vi "NI-USB6343.vi"() -> ()   [LabVIEW 2020]
doc: "test"
uses:
  LabVIEW 2020 Toolkits/toolkits_lv2020_32bit/Synchronization.llb/SynchRefs_SetGet.ctl
  LabVIEW 2020 Toolkits/VI Server Toolkit/VI Server Libraries/VI Server_SetControl.llb/VI Server_BOOL_Set.vi
  LabVIEW 2020 Toolkits/VI Server Toolkit/VI Server Libraries/VI Server_Set Controls.llb/Set STR Control.vi
  LabVIEW 2020 Toolkits/VI Server Toolkit/VI Server Libraries/VI Server_GetControl.llb/VI Server_STR_Get.vi
  LabVIEW 2020 Toolkits/VI Server Toolkit/VI Server Libraries/VI Server_GetControl.llb/VI Server_DAQmx_Device_Get.vi
  LabVIEW 2020 Toolkits/VI Server Toolkit/VI Server Toolkit LV2013.lvlib
panel:
  in  "LastAction.AddToSecuence":bool
  out "System.Message":string caption="System Message"
  in  "Help":bool
  in  "FP.Hide":bool caption="FrontPanel.Hide"
  in  "EXIT":bool
  in  "Tab.Main":T1(tab)
  in  "AI.SaveGraphToFile":bool
  in  "AI.Graph.Plots":u16(ring) items=["NI-USB6343/ai0", "NI-USB6343/ai2"]
  out "AI.WaveformGraph":waveform(dbl)[](graph) caption="Waveform Graph"
  in  "AI.MultiChannelAcquisition":bool
  in  "AI.PhysicalChannel.Include":bool
  out "AI.ActualSampleRate":dbl=1000.0 caption="Actual Sample Rate" format="%0.2f"
  out "AI.Averaged.Mesurement":dbl caption="Averaged Mesurement" format="%0.4f V"
  in  "AI.Measure":bool caption="AI:Measure"
  in  "AI.Number.Of.Samples":i32=100 caption="Number Of Samples"
  in  "AI.SampleRate":dbl=1000.0 caption="Sample Rate" format="%0.0f Hz"
  in  "AI.MinInputLimit":dbl caption="Min Input Limit" min=-10.0 max=10.0 format="%0.3f V"
  in  "AI.MaxInputLimit":dbl caption="Max Input Limit" min=-10.0 max=10.0 format="%0.3f V"
  in  "AI.TerminalConfiguration":u16(ring)=65535 caption="Terminal Configuration" items=["default"=65535, "RSE"=10083, "NRSE"=10078, "Differential"=10106, "Pseudodifferential"=12529]
  in  "AI.Sample.Mode":u16(ring)=12522 caption="Sample Mode" items=["Finite Samples"=10178, "Continuous Samples"=10123]
  in  "AI.Physical.Channel":tag="Dev1/ai0" caption="Physical Channel"
  out "AO.Update.Time":u32 caption="AO Update Time" format="%.0f msec"
  in  "AO.GenerationMode":u16(ring) caption="Generation Mode" items=["Voltage DC", "Voltage Sine Wave Generation", "Voltage Triangle Wave Generation", "Voltage Square Wave Generation", "Voltage Sawtooth Wave Generation"]
  in  "AO.Physical.Channel":tag="Dev1/ai0" caption="Physical Channel"
  in  "AO.Update":bool
  in  "AO.Output":bool caption="AO:Output"
  in  "AO.SampleMode":u16(ring) caption="Sample Mode" items=["Finite Samples"=10178, "Continious Samples"=10123]
  in  "AO.NumberOfSamples":i32=1000 caption="Number Of Samples" min=2
  in  "AO.SampleRate":dbl=1000.0 caption="Sample Rate" format="%0.1f Hz"
  in  "AO.Sample.Clock.Source":tag="OnboardClock" caption="Sample Clock Source"
  out "AO.ActualSampleRate":dbl=1000.0 caption="Actual Sample Rate" format="%0.2f"
  in  "AO.MaxVoltage":dbl=5.0 caption="Max Voltage" format="%0.3f V"
  in  "AO.MinVoltage":dbl=-5.0 caption="Min Voltage" format="%0.3f V"
  out "AO.WaveformGraph":waveform(dbl)(graph) caption="Waveform Graph"
  in  "AO.OutputVoltage":dbl(slide) caption="Amplitude" min=-10.0 max=10.0 scale=-10.0..10.0 scale format="%0.3f V"
  in  "AO.SinewaveFrequency":dbl=10.0 caption="Sinewave Frequency" format="%0.2p Hz"
  in  "DO.Port.Mask.Apply":bool caption="DO:Port.Mask.Apply"
  in  "DO.Port.Lines.31:24.Mask":u8 caption="Port&Lines 31:24" format="%08b"
  in  "DO.Port.Lines.23:16.Mask":u8 caption="Port&Lines 23:16" format="%08b"
  in  "DO.Port.Lines.15:8.Mask":u8 caption="Port&Lines 15:8" format="%08b"
  in  "DO.Port.Lines.7:0.Mask":u8 caption="Port&Lines 7:0" format="%08b"
  out "DO.Port.State.Verify":bool caption="Verified"
  out "DO.Line.State.Verify":bool caption="Verified"
  in  "DO.Line.State":bool caption="State"
  in  "DO.Line":tag="Dev1/port0/line0:7" caption="Line"
  in  "DO.Line.Update":bool caption="Update:"
  in  "DO.Port.Update":bool caption="DO:Port.Update"
  in  "DO.Port.Lines.31:24":u8 caption="Port&Lines 31:24" format="%08b"
  in  "DO.Port.Lines.23:16":u8 caption="Port&Lines 23:16" format="%08b"
  in  "DO.Port.Lines.15:8":u8 caption="Port&Lines 15:8" format="%08b"
  in  "DO.Port.Lines.7:0":u8 caption="Port&Lines 7:0" format="%08b"
  in  "DO.Port":tag="Dev1/port0/line0:7" caption="Port"
  out "DI.Line.State":bool caption="State"
  in  "DI.Port.Update":bool caption="DI:Port.Update"
  out "DI.Port.Lines.24:31":u8 caption="Port&Lines 31:24" format="%08b"
  out "DI.Port.Lines.16:23":u8 caption="Port&Lines 23:16" format="%08b"
  out "DI.Port.Lines.8:15":u8 caption="Port&Lines 15:8" format="%.0b"
  out "DI.Port.Lines.0:7":u8 caption="Port&Lines 7:0" format="%08b"
  in  "DI.Port":tag="Dev1/port0/line0:7" caption="Port"
  in  "DI.Line":tag="Dev1/port0/line0:7" caption="Line"
  in  "DI.Line.Update":bool caption="Update:"
  out "ctr3.Out.Duty Cycle.Actual":dbl caption="Ctr3: Duty Cycle Actual" format="%.2f"
  out "ctr3.Out.Frequency.Actual":dbl caption="Ctr3: Frequency Actual" format="%0.3f Hz"
  out "ctr2.Out.Duty Cycle.Actual":dbl caption="Ctr2: Duty Cycle Actual" format="%.2f"
  out "ctr2.Out.Frequency.Actual":dbl caption="Ctr2: Frequency Actual" format="%0.3f Hz"
  out "ctr1.Out.Duty Cycle.Actual":dbl caption="Ctr1: Duty Cycle Actual" format="%.2f"
  out "ctr1.Out.Frequency.Actual":dbl caption="Ctr1: Frequency Actual" format="%0.3f Hz"
  out "ctr0.Out.Duty Cycle.Actual":dbl caption="Ctr0: Duty Cycle Actual" format="%.2f"
  out "ctr0.Out.Frequency.Actual":dbl caption="Ctr0: Frequency Actual" format="%0.3f Hz"
  in  "Cntr.Out.NumberOfPulses":i32=1000 caption="Number Of Pulses" min=1
  in  "Cntr.Out.Start":bool
  in  "Cntr.Out.Sample.Mode":u16(ring)=10123 caption="Sample Mode" items=["Finite Samples"=10178, "Continuous Samples"=10123, "Hardware Timed Single Point"=12522]
  in  "Cntr.Out.Duty.Cycle":dbl=0.5 caption="Duty Cycle" format="%.2f %"
  in  "Cntr.Out.Frequency":dbl=1.0 caption="Frequency" format="%0.3f Hz"
  in  "Cntr.Out.Output.Terminal":tag="/Dev1/PFI12" caption="Output Terminal"
  in  "Cntr.Out.Channel":tag="Dev1/ctr0" caption="Channel"
  out "ctr3.In.Count":u32 caption="Count.3:"
  out "ctr2.In.Count":u32 caption="Count.2:"
  out "ctr1.In.Count":u32 caption="Count.1:"
  out "ctr0.In.Count":u32 caption="Count.0:"
  in  "Cntr.In.Start":bool
  in  "Cntr.In.IntegrationTime":u32=10 format="%.0f msec"
  in  "Cntr.In.Sample.Clock.Source":tag="PFI0" caption="Sample Clock Source"
  in  "Cntr.In.ActiveEdge":u16(ring)=10280 caption="Active Edge" items=["Rising"=10280, "Falling"=10171]
  in  "Cntr.In.Input.Terminal":tag="PFI8" caption="Input.Terminal"
  in  "Cntr.In.Channel":tag="Dev1/port0/line0:7" caption="Channel Name"
  out "TestCase.Execute.All.Done":bool
  in  "Settings.Name.Remove":bool
  in  "Settings.Name.Add":bool
  in  "Settings.Name.New":string caption="Settings Name: New"
  in  "Settings.LOAD":bool
  in  "Settings.SAVE":bool
  in  "Settings.Name":u16(ring) caption="Label" items=["AI-NEW", "AO", "Counter In", "Counter Out", "Dig I/O"]
  in  "TestCase.Execute.Step.Pause":bool
  in  "TestCase.Execute.Steps":u16(ring) caption="Test Case: Pause Before Step" items=["1", "2", "3", "4", "5", "6", "7", "8", "9", "10"]
  in  "TestCase.Execute.ABORT":bool
  in  "TestCase.Execute.Next":bool
  in  "TestCase.Execute.Pause":bool
  out "TestCase.ExecutionTime":dbl caption="Execution Time:" format="%0.3f sec"
  in  "TestCase.Execution.StepTime":u32 caption="Seq. Execution: Step Time" format="%d msec"
  in  "TestCase.Execute.All":bool
  in  "TestCase.Execute.Selected":bool
  out "TestCase.SAVE.Success":bool
  in  "TestCase.SAVE":bool
  in  "SequenceFile.Open":bool
  in  "SequenceFile":path caption="Secuence File"
  in  "TestCaseConfiguration":i32[](listbox) caption="Test Case Configuration"
  in  "TestCase.StepDescription":string caption="Step Description:"
  in  "DisableFP_OpenOnIDN_Call":bool caption="Disable FP Open\nON *IDN? Call"
  in  "DisableFP_Hide":bool caption="Disable FP Hide"
  in  "UDP.Test.String1.SendLocal":bool caption="UDP.Test.String1.Send"
  in  "ProductType":string="USB-6343 (BNC)" caption="Product Type"
  in  "VI.WindowsTitle":string caption="Windows Title"
  in  "DAQmx.Device":tag caption="DAQmx: Device"
  in  "Cont.Measurements.CycleTime":u32 caption="Continius Measurements:\nCycleTime"
  in  "UDP.Test.String2.Send":bool
  in  "UDP.Test.String2":string caption="UDP: Test String 2"
  in  "UDP.Port.BC":u16=58433 caption="UDP: Port.BC"
  in  "UDP.Port.RT":u16=58432 caption="UDP: Port.RT"
  in  "UDP.LocalPort":u16=58434 caption="UDP: Local Port"
  in  "UDP.IP.Address":string="234.5.6.7" caption="UDP: IP Address"
  in  "UDP.Test.String1.Send.ToInstr":bool caption="UDP.Test.String1.Send"
  in  "UDP.Test.String1":string caption="UDP: Test String 1"
  in  "UDP.Responce.String.Monitor":bool
  out "UDP.ExecEng.Message.String":string caption="UDP: Execution Engine Message String"
  out "error out":errorcluster={"status"=TRUE, "code"=1055, "source"="Property Node in VI Server Toolkit LV2013.lvlib:VI server_Set Control Value from String Format.vi:5200001->DMM6500_UDP_ExecEng_Instruction_APPLY.vi->DMM6500_UDP_MAIN.vi->Keithley2100.vi"}
  in  "error in":errorcluster
  # "Important Note: Analog Input configuration shall\nstart from Physical Channel selection!"
  # "Important Note: Analog Output configuration shall\nstart from Physical Channel selection!"
  # "Analog Output Configuration (Generic)"
  # "Digital Output Port\nMASK"
  # "Instructions:\n1: Active Bit; 0: Masked Bit"
  # "Digital Output"
  # "Digital Input"
  # "Counter Input"
  # "Counter Input"
  # "Counter Output"
  # "M"
  # "M"
  # "Settings"
  # "M"
  # "M"
  # "Multicast IP addresses must be in the 224.0.0.0 to 239.255.255.255 range."
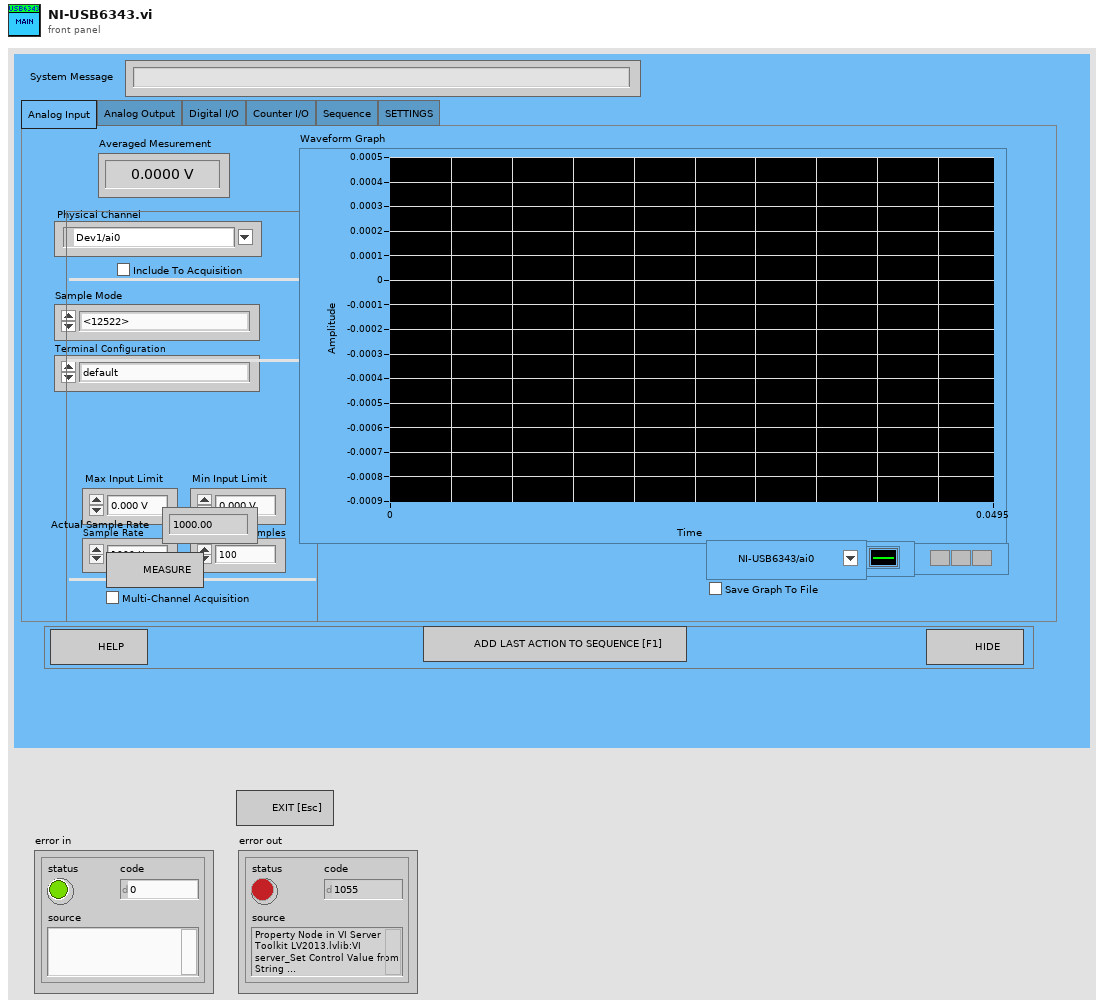
[diagram p1: front panel]
types:
  T1 = enum32{"Analog Input", "Analog Output", "Digital I/O", "Counter I/O", "Sequence", "SETTINGS"}
  T2 = typedef "VI Server_RefsCluster.ctl" = cluster{"Labels":string[], "Refs":refnum<vi>[], "VI Ref":refnum<vi>}
  T3 = typedef "SynchRefs_SetGet.ctl" = enum16{"Set", "Get"}
  T4 = enum8{"Enabled", "Disabled", "Disabled and Grayed Out"}
  T5 = cluster{"Color":u32, "PointStyle":u8, "LineStyle":u8, "Interp":u8, "LineWidth":u8, "BarPlotStyle":u8, "FillTo":i16, "XScaleIdx":u32, "YScaleIdx":u32, "Anti-Aliased":bool, "LabelFormat":u8, "TransitionType":u8, "TransitionLocation":u8, "DigitalLineStyle":u8}
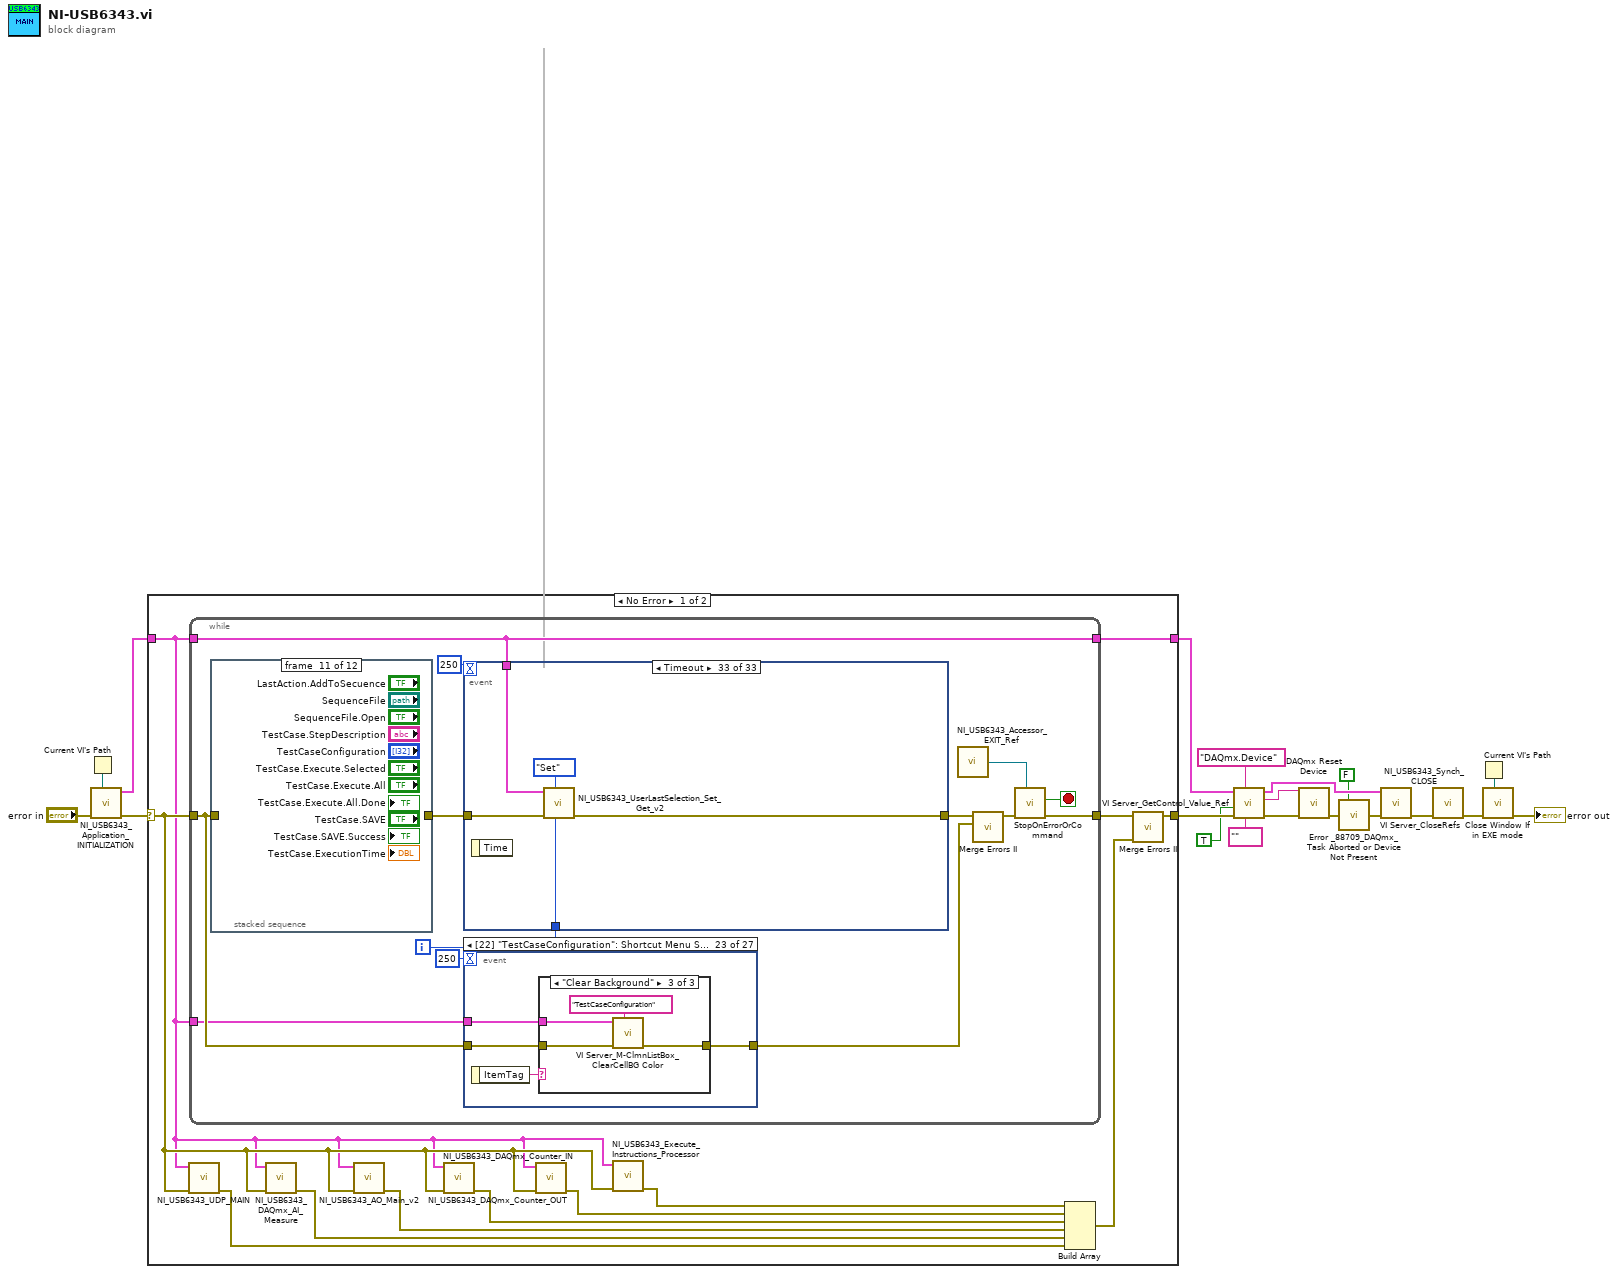
[diagram p0: block diagram]
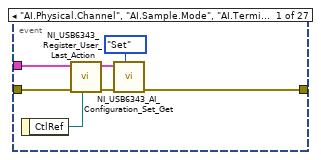
[diagram p2: hidden frame]
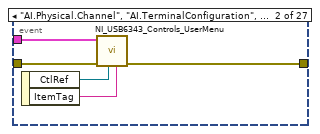
[diagram p3: hidden frame]
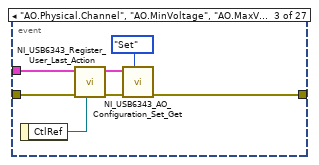
[diagram p4: hidden frame]
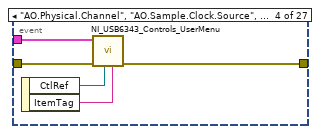
[diagram p5: hidden frame]
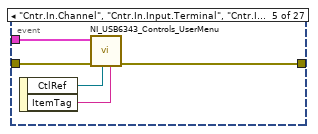
[diagram p6: hidden frame]
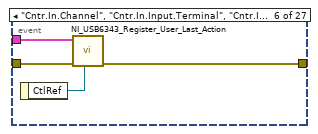
[diagram p7: hidden frame]
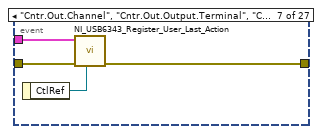
[diagram p8: hidden frame]
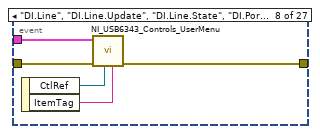
[diagram p9: hidden frame]
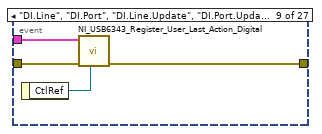
[diagram p10: hidden frame]
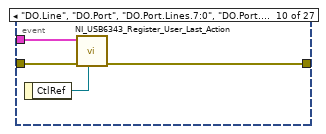
[diagram p11: hidden frame]
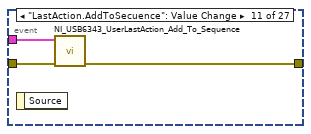
[diagram p12: hidden frame]
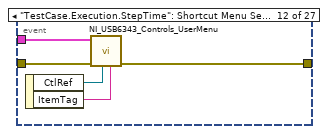
[diagram p13: hidden frame]
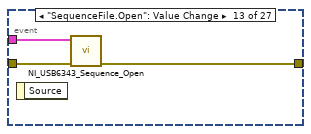
[diagram p14: hidden frame]
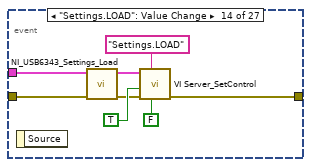
[diagram p15: hidden frame]
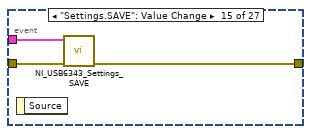
[diagram p16: hidden frame]
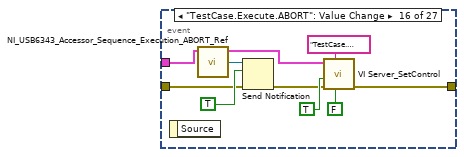
[diagram p17: hidden frame]
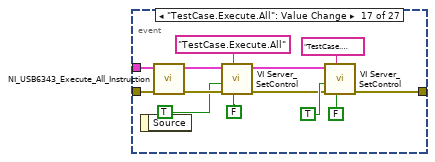
[diagram p18: hidden frame]
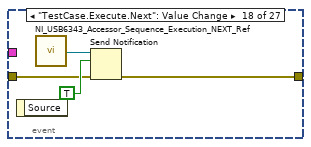
[diagram p19: hidden frame]
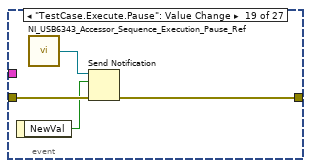
[diagram p20: hidden frame]
diagram:
  n1 = Current VI's Path() -> (path=w3:path)
  n2 = call "NI_USB6343_Application_INITIALIZATION.vi"("Top VI Path"=w3, "error in (no error)"="error in") -> ("error out"=w19:errorcluster, "VI Server Cluster.OUT"=w2:T2)  [unwired: 8 in]
  n3 = case shown="No Error" w19 {
    selector: w19 -> [w22 w407]
    tunnel: [w28 w407] -> w13
    tunnel: w2 -> [w20 w406]
    tunnel: [w31 w406] -> w11
    frame No Error {
      n4 = call "NI_USB6343_UDP_MAIN.vi"("error in (no error)"=w22, "VI Server.RefsCluster"=w20) -> ("error out"=w30:errorcluster)  [unwired: 9 in]
      n5 = while {
        tunnel: w22 -> [w36]
        tunnel: [w40] -> w29
        tunnel: w20 -> [w41]
        tunnel: [w41] -> w31
        tunnel: w20 -> [w32]
        i -> [w42]
        stop <- w39 stop-if-true
        n6 = stacked-sequence {
          tunnel: w36 -> [w405 _ _ _ _ _ _ _ _ _ _ _]
          tunnel: [w405 _ _ _ _ _ _ _ _ _ _ _] -> w44
          frame #0 {
          }
          frame #1 {
          }
          frame #2 {
          }
          frame #3 {
          }
          frame #4 {
          }
          frame #5 {
          }
          frame #6 {
          }
          frame #7 {
          }
          frame #8 {
          }
          frame #9 {
          }
          frame #10 {
          }
          frame #11 {
          }
        }
        n7 = event shown="[32] Timeout" {
          selector: _ -> [_ _ _ _ _ _ _ _ _ _ _ _ _ _ _ _ _ _ _ _ _ _ _ _ _ _ _ _ _ _ _ _ _]
          dyn-events: _ -> [_ _ _ _ _ _ _ _ _ _ _ _ _ _ _ _ _ _ _ _ _ _ _ _ _ _ _ _ _ _ _ _ _]
          timeout: 250 -> [_ _ _ _ _ _ _ _ _ _ _ _ _ _ _ _ _ _ _ _ _ _ _ _ _ _ _ _ _ _ _ _ _]
          tunnel: w44 -> [w187 w201 w204 w210 w219 w234 w241 w254 w266 w273 w276 w281 w292 w298 w304 w307 w311 w314 w318 w321 w325 w334 w341 w344 w345 w355 w357 w361 w372 w381 w390 w399 w403]
          tunnel: w42 -> [_ _ _ _ _ _ _ _ _ _ _ _ _ _ _ _ _ _ _ _ _ _ _ _ _ _ _ _ _ _ _ _ w402]
          tunnel: [w189 w199 w205 w212 w217 w232 w239 w251 w267 w271 w277 w279 w286 w297 w301 w306 w309 w312 w316 w319 w324 w331 w339 w342 w347 w350 w357 w359 w370 w379 w388 w397 w400] -> w35
          tunnel: w41 -> [w186 _ w206 w208 _ w230 w240 w253 w264 w272 w275 w280 w291 w296 w303 w305 w310 w313 _ w320 w323 _ w340 w343 _ w354 _ w358 _ w378 w387 w396 w401]
          event "AI.Physical.Channel": Value Change {
            n8 = event-data() -> ("OldVal"=w184:tag, "NewVal"=w182:tag)  [unwired: 1 in]
            n9 = call "NI_USB6343_AI_CheckPhysicalChannel.vi"("NewVal"=w182, "OldVal"=w184, "error in (no error)"=w187, "VI Server Cluster"=w186) -> ("error out"=w188:errorcluster, "AI.Settings.Update"=w183:bool, "VI Server Cluster DUP"=w185:T2)  [unwired: 5 in]
            n10 = case shown="True" w183 {
              tunnel: [w190 w193] -> w189
              tunnel: w188 -> [w190 w196]
              tunnel: w185 -> [_ w195]
              tunnel: w182 -> [_ w192]
              frame False {
              }
              frame True {
                n11 = Type Cast(x=w192) -> (*(type *) &x=w191:string)  [unwired: 1 in]
                n12 = call "NI_USB6343_AI_Configuration_Set_Get.vi"("SynchRefs.Set/Get"=SynchRefs_SetGet."Get", "error in (no error)"=w196, "VI Server Cluster"=w195) -> ("error out"=w194:errorcluster)  [unwired: 6 in, 2 out]
                n13 = property on="AI.WaveformGraph" class="WFGraph (strict)"(error in=w194, "Plot.Plot Name"=w191) -> (error out=w193:errorcluster)  [unwired: 1 in, 1 out]
              }
            }
          }
          event "AI.SaveGraphToFile": Value Change {
            n14 = event-data() -> ("NewVal"=w198:bool)  [unwired: 1 in]
            n15 = call "NI_USB6343_Accessor_AI_SaveGraphToFile_Ref.vi"() -> ("AI.SaveGraphToFile"=w200:refnum<notifier>)  [unwired: 6 in]
            n16 = Send Notification(notification=w198, notifier=w200, error in (no error)=w201) -> (error out=w199:errorcluster)  [unwired: 1 out]
          }
          event "AI.WaveformGraph": Plot Attribute Change {
            n17 = event-data() -> ("OldAttrib"=w203:T5, "NewAttrib"=w202:T5)  [unwired: 1 in]
            n18 = call "NI_USB6343_AI_Graph_PlotAttribute_ValueChanged.vi"("NewAttrib"=w202, "OldAttrib"=w203, "error in (no error)"=w204, "VI Server Cluster"=w206) -> ("error out"=w205:errorcluster)  [unwired: 7 in]
          }
          event "AO.GenerationMode": Value Change {
            n19 = event-data() -> ("NewVal"=w216:u16)  [unwired: 1 in]
            n20 = call "NI_USB6343_AO_Configuration_Set_Get.vi"("SynchRefs.Set/Get"=SynchRefs_SetGet."Set", "error in (no error)"=w210, "VI Server Cluster"=w208) -> ("error out"=w211:errorcluster, "VI Server Cluster.DUP"=w209:T2)  [unwired: 6 in, 1 out]
            n21 = call "NI_USB6343_AO_GenerationMode.vi"("AO.GenerationMode"=w216, "error in (no error)"=w211, "VI Server Cluster"=w209) -> ("error out"=w213:errorcluster)  [unwired: 7 in, 1 out]
            n22 = call "NI_USB6343_Accessor_ao_Waveform_Array_Update_Ref.vi"() -> ("ao.Waveform.Array.Update"=w215:refnum<notifier>)  [unwired: 6 in]
            n23 = Send Notification(notification=TRUE, notifier=w215, error in (no error)=w213) -> (error out=w212:errorcluster)  [unwired: 1 out]
          }
          event "AO.Output": Value Change {
            n24 = event-data() -> ("NewVal"=w218:bool)  [unwired: 1 in]
            n25 = disable-structure shown="Enabled" {
              disable-tunnel: w219 -> [w226 w227]
              disable-tunnel: w218 -> [w224 _]
              disable-tunnel: [w221 w227] -> w217
              frame Enabled {
                n26 = call "NI_USB6343_Accessor_ao0_State_Ref.vi"() -> ("ao0.State"=w225:refnum<notifier>)  [unwired: 6 in]
                n27 = Send Notification(notification=w224, notifier=w225, error in (no error)=w226) -> (error out=w222:errorcluster)  [unwired: 1 out]
                n28 = call "NI_USB6343_Accessor_ao_Waveform_Array_Update_Ref.vi"() -> ("ao.Waveform.Array.Update"=w223:refnum<notifier>)  [unwired: 6 in]
                n29 = Send Notification(notification=TRUE, notifier=w223, error in (no error)=w222) -> (error out=w221:errorcluster)  [unwired: 1 out]
              }
              frame Disabled {
              }
            }
          }
          event "AO.Physical.Channel": Value Change {
            n30 = event-data() -> ("NewVal"=w228:tag)  [unwired: 1 in]
            n31 = call "NI_USB6343_AO_Configuration_Set_Get.vi"("SynchRefs.Set/Get"=SynchRefs_SetGet."Get", "error in (no error)"=w234, "VI Server Cluster"=w230) -> ("error out"=w231:errorcluster, "VI Server Cluster.DUP"=w229:T2)  [unwired: 6 in, 1 out]
            n32 = call "NI_USB6343_AO_PhysicalChannel_UpdateGraph.vi"("AO.Physical.Channel"=w228, "error in (no error)"=w231, "VI Server Cluster"=w229) -> ("error out"=w232:errorcluster)  [unwired: 8 in]
          }
          event "AO.Sample.Clock.Source", "AO.SampleMode", "AO.SampleRate", "AO.NumberOfSamples", "AO.MaxVoltage", "AO.MinVoltage": Value Change {
            n33 = event-data() -> ()  [unwired: 1 in, 1 out]
            n34 = call "NI_USB6343_AO_ConfigurationAtributes.vi"("error in (no error)"=w241, "VI Server Cluster"=w240) -> ("error out"=w238:errorcluster)  [unwired: 8 in, 1 out]
            n35 = call "NI_USB6343_Accessor_ao0_State_Ref.vi"() -> ("ao0.State"=w236:refnum<notifier>)  [unwired: 6 in]
            n36 = Get Notifier Status(notifier=w236, error in (no error)=w238) -> (current notification=w235:bool, error out=w237:errorcluster)  [unwired: 3 out]
            n37 = case shown="True" w235 {
              tunnel: [w242 w247] -> w239
              tunnel: w237 -> [w242 w244]
              tunnel: w236 -> [_ w243]
              frame False {
              }
              frame True {
                w246 = TRUE ("notification")
                n38 = Send Notification(notification=FALSE, notifier=w243, error in (no error)=w244) -> (error out=w249:errorcluster)  [unwired: 1 out]
                n39 = call "NI_USB6343_Accessor_ao_Waveform_Array_Update_Ref.vi"() -> ("ao.Waveform.Array.Update"=w250:refnum<notifier>)  [unwired: 6 in]
                n40 = Send Notification(notification=w246, notifier=w250, error in (no error)=w249) -> (error out=w248:errorcluster)  [unwired: 1 out]
                n41 = Send Notification(notification=w246, notifier=w243, error in (no error)=w248) -> (error out=w247:errorcluster)  [unwired: 1 out]
              }
            }
          }
          event "AO.SinewaveFrequency", "AO.OutputVoltage": Value Change {
            n42 = event-data() -> ()  [unwired: 1 in, 4 out]
            n43 = call "VI Server_CycleEventBySignalingValue.vi"("Label"="AO.GenerationMode", "error in"=w254, "VI Server.RefsCluster"=w253) -> ("error out"=w251:errorcluster)  [unwired: 7 in, 1 out]
          }
          event "AO.Update": Value Change {
            w257 = TRUE ("Single Instance (T)")
            n44 = event-data() -> ()  [unwired: 1 in, 1 out]
            n45 = call "VI Server_Get Text Ring Selection.vi"("Label"="AO.GenerationMode", "error in"=w266, "Single Instance (T)"=w257, "VI Server Cluster"=w264) -> ("error out"=w262:errorcluster, "VI Server Custer.DUP"=w263:T2, "Value"=w261:u16)  [unwired: 2 in, 3 out]
            n46 = call "NI_USB6343_AO_GenerationMode.vi"("AO.GenerationMode"=w261, "error in (no error)"=w262, "VI Server Cluster"=w263) -> ("error out"=w260:errorcluster, "VI Server Cluster.DUP"=w258:T2)  [unwired: 7 in]
            n47 = call-poly "VI Server_SetControl.vi"("Data"=FALSE, "Control.Label"="AO.Update" ("Label"), "error in"=w260, "SingleInstance"=w257, "VI Server.RefsCluster"=w258) -> ("error out"=w259:errorcluster)  [unwired: 4 in, 2 out]
            n48 = call "NI_USB6343_Accessor_ao_Waveform_Array_Update_Ref.vi"() -> ("ao.Waveform.Array.Update"=w269:refnum<notifier>)  [unwired: 6 in]
            n49 = Send Notification(notification=TRUE, notifier=w269, error in (no error)=w259) -> (error out=w267:errorcluster)  [unwired: 1 out]
          }
          event "Cntr.In.Channel": Value Change {
            n50 = event-data() -> ("NewVal"=w270:tag)  [unwired: 1 in]
            n51 = call "NI-USB6343_Counter_IN_GetStateFromFile.vi"("Counter.IN.Channel"=w270, "error in (no error)"=w273, "VI Server Cluster"=w272) -> ("error out"=w271:errorcluster)  [unwired: 7 in, 1 out]
          }
          event "Cntr.In.Start": Value Change {
            n52 = event-data() -> ("NewVal"=w274:bool)  [unwired: 1 in]
            n53 = call "NI-USB6343_Counter_IN_SaveStateToFile.vi"("Cntr.In.Start"=w274, "error in (no error)"=w276, "VI Server Cluster"=w275) -> ("error out"=w277:errorcluster)  [unwired: 7 in, 1 out]
          }
          event "Cntr.Out.Channel": Value Change {
            n54 = event-data() -> ("NewVal"=w282:tag, "OldVal"=w278:tag)  [unwired: 1 in]
            n55 = call "NI-USB6343_Counter_OUT_GetStateFromFile.vi"("Counter.OUT.Channel.Old"=w278, "Counter.OUT.Channel.New"=w282, "error in (no error)"=w281, "VI Server Cluster"=w280) -> ("error out"=w279:errorcluster)  [unwired: 6 in, 1 out]
          }
          event "Cntr.Out.Sample.Mode": Value Change {
            n56 = event-data() -> ()  [unwired: 1 in, 1 out]
            n57 = call "VI Server_Get Text Ring Selection.vi"("Label"="Cntr.Out.Sample.Mode", "error in"=w292, "Single Instance (T)"=TRUE, "VI Server Cluster"=w291) -> ("error out"=w287:errorcluster, "Selection"=w288:string, "VI Server Custer.DUP"=w285:T2)  [unwired: 2 in, 3 out]
            n58 = case shown="\"Finite Samples\"" w288 {
              tunnel: [T4."Disabled and Grayed Out" ("Disabled") T4."Enabled" ("Disabled")] -> w284
              frame "Continuous Samples", Default {
              }
              frame "Finite Samples" {
              }
            }
            n59 = call "VI Server_Enable_Disable.vi"("Disabled"=w284, "Label"="Cntr.Out.NumberOfPulses", "error in"=w287, "VI Server Cluster"=w285) -> ("error out"=w286:errorcluster)  [unwired: 5 in, 2 out]
          }
          event "Cntr.Out.Start": Value Change {
            n60 = event-data() -> ("NewVal"=w295:bool)  [unwired: 1 in]
            n61 = call "NI-USB6343_Counter_OUT_SaveStateToFile.vi"("Cntr.In.Start"=w295, "error in (no error)"=w298, "VI Server Cluster"=w296) -> ("error out"=w297:errorcluster)  [unwired: 7 in, 1 out]
          }
          event "DAQmx.Device": Value Change {
            n62 = event-data() -> ("NewVal"=w299:tag)  [unwired: 1 in]
            n63 = call "NI_USB6343_DAQmx_LimitPhysicalChannelsToDevice.vi"("error in (no error)"=w304, "VI Server Cluster"=w303) -> ("error out"=w302:errorcluster, "VI Server Cluster.DUP"=w300:T2)  [unwired: 7 in, 1 out]
            n64 = call "NI_USB6343_DAQmx_DeviceName_Changed_UpdateSet_Get_Sections.vi"("DAQmx.Device"=w299, "error in (no error)"=w302, "VI Server Cluster"=w300) -> ("error out"=w301:errorcluster)  [unwired: 8 in]
          }
          event "DI.Line.Update": Value Change {
            n65 = event-data() -> ()  [unwired: 1 in, 1 out]
            n66 = call "NI_USB6343_Digital_Input_Line_Update.vi"("error in (no error)"=w307, "VI Server Cluster"=w305) -> ("error out"=w306:errorcluster)  [unwired: 9 in]
          }
          event "DI.Port": Value Change {
            n67 = event-data() -> ("NewVal"=w308:tag)  [unwired: 1 in]
            n68 = call "NI_USB6343_DI_Port_ValueChanged.vi"("DI.Port"=w308, "error in (no error)"=w311, "VI Server Cluster"=w310) -> ("error out"=w309:errorcluster)  [unwired: 8 in]
          }
          event "DI.Port.Update": Value Change {
            n69 = event-data() -> ()  [unwired: 1 in, 1 out]
            n70 = call "NI_USB6343_DI_Port_Update.vi"("error in (no error)"=w314, "VI Server Cluster"=w313) -> ("error out"=w312:errorcluster)  [unwired: 9 in]
          }
          event "DisableFP_Hide": Value Change {
            n71 = event-data() -> ("NewVal"=w315:bool)  [unwired: 1 in]
            n72 = call "NI_USB6343_Accessor_DisableFP_Hide_Ref.vi"() -> ("DisableFP_Hide"=w317:refnum<notifier>)  [unwired: 6 in]
            n73 = Send Notification(notification=w315, notifier=w317, error in (no error)=w318) -> (error out=w316:errorcluster)  [unwired: 1 out]
          }
          event "DO.Line.Update": Value Change {
            n74 = event-data() -> ()  [unwired: 1 in, 1 out]
            n75 = call "NI_USB6343_Digital_Output_Line_Update.vi"("error in (no error)"=w321, "VI Server Cluster"=w320) -> ("error out"=w319:errorcluster)  [unwired: 9 in]
          }
          event "DO.Port": Value Change {
            n76 = event-data() -> ("NewVal"=w322:tag)  [unwired: 1 in]
            n77 = call "NI_USB6343_DO_Port_ValueChanged.vi"("DO.Port"=w322, "error in (no error)"=w325, "VI Server Cluster"=w323) -> ("error out"=w324:errorcluster)  [unwired: 8 in]
          }
          event "DO.Port.Lines.7:0", "DO.Port.Lines.15:8", "DO.Port.Lines.23:16", "DO.Port.Lines.31:24", "DO.Port.Lines.7:0.Mask", "DO.Port.Lines.15:8.Mask", "DO.Port.Lines.23:16.Mask", "DO.Port.Lines.31:24.Mask", "DI.Port.Lines.0:7", "DI.Port.Lines.8:15", "DI.Port.Lines.16:23", "DI.Port.Lines.24:31": Mouse Down {
            n78 = event-data() -> ("CtlRef"=w333:refnum<vi>)  [unwired: 1 in]
            n79 = property class="DigNum (strict)"(reference=w333, error in=w334) -> (reference out=w330:refnum<vi>, error out=w332:errorcluster, "FormatString"=w327:string)
            n80 = Match Pattern(string=w327, regular expression="[0-9]+") -> (after substring=w326:string)  [unwired: 1 in, 3 out]
            n81 = case shown="\"b\", Default" w326 {
              tunnel: ["%.0f" "%02x" "%02o" "%08b"] -> w329
              frame "f" {
              }
              frame "x" {
              }
              frame "o" {
              }
              frame "b", Default {
              }
            }
            n82 = property class="DigNum (strict)"(reference=w330, error in=w332, "FormatString"=w329) -> (error out=w331:errorcluster)  [unwired: 1 out]
          }
          event "DO.Port.Mask.Apply": Value Change {
            n83 = event-data() -> ()  [unwired: 1 in, 1 out]
            n84 = call "NI_USB6343_DO_Port_Mask_Apply.vi"("error in (no error)"=w341, "VI Server Cluster"=w340) -> ("error out"=w339:errorcluster)  [unwired: 9 in]
          }
          event "DO.Port.Update": Value Change {
            n85 = event-data() -> ()  [unwired: 1 in, 1 out]
            n86 = call "NI_USB6343_DO_Port_Update.vi"("error in (no error)"=w344, "VI Server Cluster"=w343) -> ("error out"=w342:errorcluster)  [unwired: 9 in]
          }
          event "EXIT": Value Change {
            n87 = event-data() -> ()  [unwired: 1 in, 1 out]
            n88 = call "NI_USB6343_Accessor_EXIT_Ref.vi"() -> ("EXIT"=w348:refnum<notifier>)  [unwired: 6 in]
            n89 = Send Notification(notification=TRUE, notifier=w348, error in (no error)=w345) -> (error out=w347:errorcluster)  [unwired: 1 out]
          }
          event "FP.Hide": Value Change {
            n90 = event-data() -> ("NewVal"=w349:bool)  [unwired: 1 in]
            n91 = call "NI_USB6343_Accessor_FP_State_Ref.vi"() -> ("FP.State"=w353:refnum<notifier>)  [unwired: 6 in]
            n92 = call "ExecEng_InstrumentsFrontPanel_Hide_Show.vi"("FP.Hide/Show"=w349, "FP.State"=w353, "error in (no error)"=w355, "VI Server Cluster"=w354) -> ("error out"=w351:errorcluster, "VI Server Cluster DUP"=w352:T2)  [unwired: 6 in]
            n93 = call "NI_USB6343_FP_Hide_SendMessageToExecEng.vi"("FP.Open"=w349, "error in (no error)"=w351, "VI Server Cluster"=w352) -> ("error out"=w350:errorcluster)  [unwired: 8 in]
          }
          event "Help": Value Change {
            n94 = event-data() -> ("NewVal"=w356:bool)  [unwired: 1 in]
            n95 = Control Help Window(1:w356) -> ()  [unwired: 1 in]
          }
          event "UDP.ExecEng.Message.String": Shortcut Menu Selection (User) {
            n96 = event-data() -> ("ItemTag"=w360:string)  [unwired: 1 in]
            n97 = case shown="\"Clear Indicator\"" w360 {
              tunnel: w361 -> [w362 w368]
              tunnel: [w362 w367] -> w359
              tunnel: w358 -> [_ w366]
              frame "", Default {
              }
              frame "Clear Indicator" {
                n98 = call-poly "VI Server_Set Control Value.vi"("New Value"="", "Label"="UDP.ExecEng.Message.String" ("Control.Label"), "error in"=w368, "Single Instance (T)"=TRUE ("SingleInstance"), "VI Server Cluster"=w366) -> ("error out"=w367:errorcluster)  [unwired: 4 in, 2 out]
              }
            }
          }
          event "UDP.Responce.String.Monitor": Value Change {
            n99 = event-data() -> ("NewVal"=w369:bool)  [unwired: 1 in]
            n100 = call "NI_USB6343_Accessor_UDP_Responce_String_Monitor_Ref.vi"() -> ("UDP.ExecEng.Command.String.Monitor"=w371:refnum<notifier>)  [unwired: 6 in]
            n101 = Send Notification(notification=w369, notifier=w371, error in (no error)=w372) -> (error out=w370:errorcluster)  [unwired: 1 out]
          }
          event "UDP.Test.String1.Send.ToInstr": Value Change {
            n102 = event-data() -> ()  [unwired: 1 in, 1 out]
            n103 = call-poly "VI Server_GetControl_Value_Ref.vi"("DataType"="", "Control.Label"="UDP.Test.String1", "error in"=w381, "SingleInstance"=TRUE, "VI Server.RefsCluster"=w378) -> ("error out"=w380:errorcluster, "Value"=w373:string)  [unwired: 3 in, 2 out]
            n104 = call "NI_USB6343_Accessor_UDP_Instrument_Responce_Ref.vi"() -> ("UDP.Instrument.Responce.Q"=w374:refnum<queue>)  [unwired: 6 in]
            n105 = Enqueue Element(queue=w374, element=w373, error in (no error)=w380) -> (error out=w379:errorcluster)  [unwired: 1 in, 2 out]
          }
          event "UDP.Test.String1.SendLocal": Value Change {
            n106 = event-data() -> ()  [unwired: 1 in, 1 out]
            n107 = call-poly "VI Server_GetControl_Value_Ref.vi"("DataType"="", "Control.Label"="UDP.Test.String1", "error in"=w390, "SingleInstance"=TRUE, "VI Server.RefsCluster"=w387) -> ("error out"=w389:errorcluster, "Value"=w383:string)  [unwired: 3 in, 2 out]
            n108 = call "NI_USB6343_Accessor_UDP_ExecEng_Instruction_Q_Ref.vi"() -> ("UDP.ExecEng.Instruction.Q"=w382:refnum<queue>)  [unwired: 6 in]
            n109 = Enqueue Element(queue=w382, element=w383, error in (no error)=w389) -> (error out=w388:errorcluster)  [unwired: 1 in, 2 out]
          }
          event "UDP.Test.String2.Send": Value Change {
            n110 = event-data() -> ()  [unwired: 1 in, 1 out]
            n111 = call-poly "VI Server_GetControl_Value_Ref.vi"("DataType"="", "Control.Label"="UDP.Test.String2", "error in"=w399, "SingleInstance"=TRUE, "VI Server.RefsCluster"=w396) -> ("error out"=w398:errorcluster, "Value"=w391:string)  [unwired: 3 in, 2 out]
            n112 = call "NI_USB6343_Accessor_UDP_Instrument_Responce_Ref.vi"() -> ("UDP.Instrument.Responce.Q"=w392:refnum<queue>)  [unwired: 6 in]
            n113 = Enqueue Element(queue=w392, element=w391, error in (no error)=w398) -> (error out=w397:errorcluster)  [unwired: 1 in, 2 out]
          }
          event Timeout {
            n114 = event-data() -> ()  [unwired: 1 in, 1 out]
            n115 = call "NI_USB6343_UserLastSelection_Set_Get_v2.vi"("LoopCounter"=w402, "SynchRefs.Set/Get"=SynchRefs_SetGet."Set", "error in"=w403, "VI Server.RefsCluster"=w401) -> ("error out"=w400:errorcluster)  [unwired: 6 in, 1 out]
          }
        }
        n116 = event shown="[22] \"TestCaseConfiguration\": Shortcut Menu Selection (User)" {
          selector: _ -> [_ _ _ _ _ _ _ _ _ _ _ _ _ _ _ _ _ _ _ _ _ _ _ _ _ _ _]
          dyn-events: _ -> [_ _ _ _ _ _ _ _ _ _ _ _ _ _ _ _ _ _ _ _ _ _ _ _ _ _ _]
          timeout: 250 -> [_ _ _ _ _ _ _ _ _ _ _ _ _ _ _ _ _ _ _ _ _ _ _ _ _ _ _]
          tunnel: w36 -> [w51 w56 w63 w67 w72 w77 w81 w85 w90 w94 w97 w101 w105 w108 w116 w123 w138 w140 w145 w149 w152 w156 w159 w174 w175 w180 w181]
          tunnel: [w45 w55 w59 w66 w71 w76 w80 w84 w88 w93 w96 w102 w103 w106 w114 w118 w126 w139 w144 w147 w151 w154 w158 w172 w176 w178 w181] -> w33
          tunnel: w32 -> [w49 w54 w62 w68 w73 w74 w78 w86 w89 w91 w95 w98 w104 w107 w115 w117 w137 _ _ w148 _ w155 w157 w173 w177 w179 _]
          event "AI.Physical.Channel", "AI.Sample.Mode", "AI.TerminalConfiguration", "AI.MaxInputLimit", "AI.MinInputLimit", "AI.SampleRate", "AI.Number.Of.Samples", "AI.MultiChannelAcquisition", "AI.Measure", "AI.PhysicalChannel.Include": Value Change {
            n117 = event-data() -> ("CtlRef"=w50:refnum<vi>)  [unwired: 1 in]
            n118 = call "NI_USB6343_Register_User_Last_Action.vi"("CtlRef"=w50, "error in (no error)"=w51, "VI Server Cluster"=w49) -> ("error out"=w46:errorcluster, "VI Server Cluster.DUP"=w47:T2)  [unwired: 7 in]
            n119 = call "NI_USB6343_AI_Configuration_Set_Get.vi"("SynchRefs.Set/Get"=SynchRefs_SetGet."Set", "error in (no error)"=w46, "VI Server Cluster"=w47) -> ("error out"=w45:errorcluster)  [unwired: 6 in, 2 out]
          }
          event "AI.Physical.Channel", "AI.TerminalConfiguration", "AI.Sample.Mode", "AI.MaxInputLimit", "AI.MinInputLimit", "AI.SampleRate", "AI.Number.Of.Samples", "AI.Measure", "AI.MultiChannelAcquisition", "AI.PhysicalChannel.Include", "TestCase.Execute.All": Shortcut Menu Selection (User) {
            n120 = event-data() -> ("CtlRef"=w53:refnum<vi>, "ItemTag"=w52:string)  [unwired: 1 in]
            n121 = call "NI_USB6343_Controls_UserMenu.vi"("ItemTag"=w52, "Control Ref"=w53, "error in (no error)"=w56, "VI Server Cluster"=w54) -> ("error out"=w55:errorcluster)  [unwired: 7 in]
          }
          event "AO.Physical.Channel", "AO.MinVoltage", "AO.MaxVoltage", "AO.Sample.Clock.Source", "AO.SampleRate", "AO.NumberOfSamples", "AO.GenerationMode", "AO.SinewaveFrequency", "AO.SampleMode", "AO.OutputVoltage": Value Change {
            n122 = event-data() -> ("CtlRef"=w61:refnum<vi>)  [unwired: 1 in]
            n123 = call "NI_USB6343_Register_User_Last_Action.vi"("CtlRef"=w61, "error in (no error)"=w63, "VI Server Cluster"=w62) -> ("error out"=w60:errorcluster, "VI Server Cluster.DUP"=w58:T2)  [unwired: 7 in]
            n124 = call "NI_USB6343_AO_Configuration_Set_Get.vi"("SynchRefs.Set/Get"=SynchRefs_SetGet."Set", "error in (no error)"=w60, "VI Server Cluster"=w58) -> ("error out"=w59:errorcluster)  [unwired: 6 in, 2 out]
          }
          event "AO.Physical.Channel", "AO.Sample.Clock.Source", "AO.NumberOfSamples", "AO.GenerationMode", "AO.MaxVoltage", "AO.MinVoltage", "AO.SampleRate", "AO.OutputVoltage", "AO.SinewaveFrequency", "AO.Update", "AO.Output": Shortcut Menu Selection (User) {
            n125 = event-data() -> ("CtlRef"=w65:refnum<vi>, "ItemTag"=w64:string)  [unwired: 1 in]
            n126 = call "NI_USB6343_Controls_UserMenu.vi"("ItemTag"=w64, "Control Ref"=w65, "error in (no error)"=w67, "VI Server Cluster"=w68) -> ("error out"=w66:errorcluster)  [unwired: 7 in]
          }
          event "Cntr.In.Channel", "Cntr.In.Input.Terminal", "Cntr.In.ActiveEdge", "Cntr.In.Sample.Clock.Source", "Cntr.In.IntegrationTime", "Cntr.In.Start", "Cntr.Out.Channel", "Cntr.Out.Output.Terminal", "Cntr.Out.Frequency", "Cntr.Out.Duty.Cycle", "Cntr.Out.Sample.Mode", "Cntr.Out.Start", "Cntr.Out.NumberOfPulses": Shortcut Menu Selection (User) {
            n127 = event-data() -> ("CtlRef"=w70:refnum<vi>, "ItemTag"=w69:string)  [unwired: 1 in]
            n128 = call "NI_USB6343_Controls_UserMenu.vi"("ItemTag"=w69, "Control Ref"=w70, "error in (no error)"=w72, "VI Server Cluster"=w73) -> ("error out"=w71:errorcluster)  [unwired: 7 in]
          }
          event "Cntr.In.Channel", "Cntr.In.Input.Terminal", "Cntr.In.ActiveEdge", "Cntr.In.Sample.Clock.Source", "Cntr.In.IntegrationTime": Value Change {
            n129 = event-data() -> ("CtlRef"=w75:refnum<vi>)  [unwired: 1 in]
            n130 = call "NI_USB6343_Register_User_Last_Action.vi"("CtlRef"=w75, "error in (no error)"=w77, "VI Server Cluster"=w74) -> ("error out"=w76:errorcluster)  [unwired: 7 in, 1 out]
          }
          event "Cntr.Out.Channel", "Cntr.Out.Output.Terminal", "Cntr.Out.Frequency", "Cntr.Out.Duty.Cycle", "Cntr.Out.Sample.Mode", "Cntr.Out.NumberOfPulses": Value Change {
            n131 = event-data() -> ("CtlRef"=w79:refnum<vi>)  [unwired: 1 in]
            n132 = call "NI_USB6343_Register_User_Last_Action.vi"("CtlRef"=w79, "error in (no error)"=w81, "VI Server Cluster"=w78) -> ("error out"=w80:errorcluster)  [unwired: 7 in, 1 out]
          }
          event "DI.Line", "DI.Line.Update", "DI.Line.State", "DI.Port", "DI.Port.Lines.0:7", "DI.Port.Lines.8:15", "DI.Port.Lines.16:23", "DI.Port.Lines.24:31", "DI.Port.Update", "DO.Line.Update", "DO.Line", "DO.Line.State", "DO.Line.State.Verify", "DO.Port", "DO.Port.Lines.7:0", "DO.Port.Lines.15:8", "DO.Port.Lines.23:16", "DO.Port.Lines.31:24", "DO.Port.Update", "DO.Port.State.Verify", "DO.Port.Lines.7:0.Mask", "DO.Port.Lines.15:8.Mask", "DO.Port.Lines.23:16.Mask", "DO.Port.Lines.31:24.Mask", "DO.Port.Mask.Apply": Shortcut Menu Selection (User) {
            n133 = event-data() -> ("CtlRef"=w83:refnum<vi>, "ItemTag"=w82:string)  [unwired: 1 in]
            n134 = call "NI_USB6343_Controls_UserMenu.vi"("ItemTag"=w82, "Control Ref"=w83, "error in (no error)"=w85, "VI Server Cluster"=w86) -> ("error out"=w84:errorcluster)  [unwired: 7 in]
          }
          event "DI.Line", "DI.Port", "DI.Line.Update", "DI.Port.Update": Value Change {
            n135 = event-data() -> ("CtlRef"=w87:refnum<vi>)  [unwired: 1 in]
            n136 = call "NI_USB6343_Register_User_Last_Action_Digital.vi"("CtlRef"=w87, "error in (no error)"=w90, "VI Server Cluster"=w89) -> ("error out"=w88:errorcluster)  [unwired: 8 in]
          }
          event "DO.Line", "DO.Port", "DO.Port.Lines.7:0", "DO.Port.Lines.15:8", "DO.Port.Lines.23:16", "DO.Port.Lines.31:24", "DO.Port.Lines.7:0.Mask", "DO.Port.Lines.15:8.Mask", "DO.Port.Lines.23:16.Mask", "DO.Port.Lines.31:24.Mask", "DO.Port.Update", "DO.Line.Update": Value Change {
            n137 = event-data() -> ("CtlRef"=w92:refnum<vi>)  [unwired: 1 in]
            n138 = call "NI_USB6343_Register_User_Last_Action.vi"("CtlRef"=w92, "error in (no error)"=w94, "VI Server Cluster"=w91) -> ("error out"=w93:errorcluster)  [unwired: 7 in, 1 out]
          }
          event "LastAction.AddToSecuence": Value Change {
            n139 = event-data() -> ()  [unwired: 1 in, 1 out]
            n140 = call "NI_USB6343_UserLastAction_Add_To_Sequence.vi"("error in (no error)"=w97, "VI Server Cluster"=w95) -> ("error out"=w96:errorcluster)  [unwired: 9 in]
          }
          event "TestCase.Execution.StepTime": Shortcut Menu Selection (User) {
            n141 = event-data() -> ("CtlRef"=w100:refnum<vi>, "ItemTag"=w99:string)  [unwired: 1 in]
            n142 = call "NI_USB6343_Controls_UserMenu.vi"("ItemTag"=w99, "Control Ref"=w100, "error in (no error)"=w101, "VI Server Cluster"=w98) -> ("error out"=w102:errorcluster)  [unwired: 7 in]
          }
          event "SequenceFile.Open": Value Change {
            n143 = event-data() -> ()  [unwired: 1 in, 1 out]
            n144 = call "NI_USB6343_Sequence_Open.vi"("error in (no error)"=w105, "VI Server Cluster"=w104) -> ("error out"=w103:errorcluster)  [unwired: 9 in]
          }
          event "Settings.LOAD": Value Change {
            n145 = event-data() -> ()  [unwired: 1 in, 1 out]
            n146 = call "NI_USB6343_Settings_Load.vi"("error in"=w108, "VI Server.RefsCluster"=w107) -> ("error out"=w110:errorcluster, "VI Server.RefsCluster.DUP"=w109:T2)  [unwired: 8 in]
            n147 = call-poly "VI Server_SetControl.vi"("Data"=FALSE, "Control.Label"="Settings.LOAD", "error in"=w110, "SingleInstance"=TRUE, "VI Server.RefsCluster"=w109) -> ("error out"=w106:errorcluster)  [unwired: 4 in, 2 out]
          }
          event "Settings.SAVE": Value Change {
            n148 = event-data() -> ()  [unwired: 1 in, 1 out]
            n149 = call "NI_USB6343_Settings_SAVE.vi"("error in"=w116, "VI Server.RefsCluster"=w115) -> ("error out"=w114:errorcluster)  [unwired: 8 in, 1 out]
          }
          event "TestCase.Execute.ABORT": Value Change {
            n150 = event-data() -> ()  [unwired: 1 in, 1 out]
            n151 = call "NI_USB6343_Accessor_Sequence_Execution_ABORT_Ref.vi"() -> ("SequenceExecution.ABORT"=w124:refnum<notifier>)  [unwired: 6 in]
            n152 = Send Notification(notification=TRUE, notifier=w124, error in (no error)=w123) -> (error out=w119:errorcluster)  [unwired: 1 out]
            n153 = call-poly "VI Server_SetControl.vi"("Data"=FALSE, "Control.Label"="TestCase.Execute.All.Done" ("Label"), "error in"=w119, "SingleInstance"=TRUE, "VI Server.RefsCluster"=w117) -> ("error out"=w118:errorcluster)  [unwired: 4 in, 2 out]
          }
          event "TestCase.Execute.All": Value Change {
            n154 = event-data() -> ()  [unwired: 1 in, 1 out]
            n155 = call "NI_USB6343_Execute_All_Instruction.vi"("error in (no error)"=w138, "VI Server Cluster"=w137) -> ("error out"=w136:errorcluster, "VI Server Cluster.DUP"=w135:T2)  [unwired: 8 in]
            n156 = call-poly "VI Server_SetControl.vi"("Data"=FALSE, "Control.Label"="TestCase.Execute.All", "error in"=w136, "SingleInstance"=TRUE, "VI Server.RefsCluster"=w135) -> ("error out"=w127:errorcluster, "VI Server.RefsCluster.DUP"=w128:T2)  [unwired: 4 in, 1 out]
            n157 = call-poly "VI Server_SetControl.vi"("Data"=FALSE, "Control.Label"="TestCase.Execute.All.Done" ("Label"), "error in"=w127, "SingleInstance"=TRUE, "VI Server.RefsCluster"=w128) -> ("error out"=w126:errorcluster)  [unwired: 4 in, 2 out]
          }
          event "TestCase.Execute.Next": Value Change {
            n158 = event-data() -> ()  [unwired: 1 in, 1 out]
            n159 = call "NI_USB6343_Accessor_Sequence_Execution_NEXT_Ref.vi"() -> ("SequenceExecution.NEXT"=w142:refnum<notifier>)  [unwired: 6 in]
            n160 = Send Notification(notification=TRUE, notifier=w142, error in (no error)=w140) -> (error out=w139:errorcluster)  [unwired: 1 out]
          }
          event "TestCase.Execute.Pause": Value Change {
            n161 = event-data() -> ("NewVal"=w143:bool)  [unwired: 1 in]
            n162 = call "NI_USB6343_Accessor_Sequence_Execution_Pause_Ref.vi"() -> ("SequenceExecution.PAUSE"=w146:refnum<notifier>)  [unwired: 6 in]
            n163 = Send Notification(notification=w143, notifier=w146, error in (no error)=w145) -> (error out=w144:errorcluster)  [unwired: 1 out]
          }
          event "TestCase.Execute.Selected": Value Change {
            n164 = event-data() -> ()  [unwired: 1 in, 1 out]
            n165 = call "NI_USB6343_ExecuteSelectedInstruction.vi"("error in (no error)"=w149, "VI Server Cluster"=w148) -> ("error out"=w147:errorcluster)  [unwired: 9 in]
          }
          event "TestCase.Execute.Step.Pause": Value Change {
            n166 = event-data() -> ("NewVal"=w150:bool)  [unwired: 1 in]
            n167 = call "NI_USB6343_TestCase_Execution_Pause_Ref.vi"() -> ("SequenceExecution.StepPAUSE"=w153:refnum<notifier>)  [unwired: 6 in]
            n168 = Send Notification(notification=w150, notifier=w153, error in (no error)=w152) -> (error out=w151:errorcluster)  [unwired: 1 out]
          }
          event "TestCase.SAVE": Value Change {
            n169 = event-data() -> ()  [unwired: 1 in, 1 out]
            n170 = call "ExecEng_InstrGeneric_Sequence_Save.vi"("error in (no error)"=w156, "VI Server Cluster"=w155) -> ("error out"=w154:errorcluster)  [unwired: 9 in]
          }
          event "TestCaseConfiguration": Shortcut Menu Selection (User) {
            n171 = event-data() -> ("ItemTag"=w160:string)  [unwired: 1 in]
            n172 = case shown="\"Clear Background\"" w160 {
              tunnel: w159 -> [w161 w167 w170]
              tunnel: [w161 w166 w169] -> w158
              tunnel: w157 -> [_ w163 w168]
              frame "False", Default {
              }
              frame "Clear Table" {
                n173 = call "VI Server_M_ClmnListBox_ItemNames_SET.vi"("Item Names"=string[][] [], "Label"="TestCaseConfiguration", "error in"=w167, "SingleInstance"=TRUE, "VI Server.RefsCluster"=w163) -> ("error out"=w166:errorcluster)  [unwired: 4 in, 2 out]
              }
              frame "Clear Background" {
                n174 = call "VI Server_M-ClmnListBox_ClearCellBG Color.vi"("Label"="TestCaseConfiguration", "error in"=w170, "VI Server Cluster"=w168) -> ("error out"=w169:errorcluster)  [unwired: 7 in, 1 out]
              }
            }
          }
          event "TestCaseConfiguration": Value Change {
            n175 = event-data() -> ()  [unwired: 1 in, 1 out]
            n176 = call "NI_USB6343_TestCase_Configuration_ValueChanged.vi"("error in"=w174, "VI Server.RefsCluster"=w173) -> ("error out"=w172:errorcluster)  [unwired: 8 in, 1 out]
          }
          event "Settings.Name.Add": Value Change {
            n177 = event-data() -> ()  [unwired: 1 in, 1 out]
            n178 = call "NI_USB6343_Sequence_AddNewSettingsLabel.vi"("error in (no error)"=w175, "VI Server Cluster"=w177) -> ("error out"=w176:errorcluster)  [unwired: 9 in]
          }
          event "Settings.Name.Remove": Value Change {
            n179 = event-data() -> ()  [unwired: 1 in, 1 out]
            n180 = call "NI_USB6343_Sequence_RemoveSettingsLabel.vi"("error in (no error)"=w180, "VI Server Cluster"=w179) -> ("error out"=w178:errorcluster)  [unwired: 9 in]
          }
          event Timeout {
            n181 = event-data() -> ()  [unwired: 1 in, 1 out]
          }
        }
        n182 = call "NI_USB6343_Accessor_EXIT_Ref.vi"() -> ("EXIT"=w38:refnum<notifier>)  [unwired: 6 in]
        n183 = call "Merge Errors II.vi"("error in 2 (no error)"=w33, "error in 1 (no error)"=w35) -> ("error out.DUP"=w34:errorcluster)  [unwired: 4 in, 1 out]
        n184 = call "StopOnErrorOrCommand.vi"("STOP"=w38, "error in (no error)"=w34) -> ("error out"=w40:errorcluster, "STOP"=w39:bool)  [unwired: 8 in]
      }
      n185 = call "NI_USB6343_DAQmx_AI_Measure.vi"("error in (no error)"=w22, "VI Server Cluster"=w20) -> ("error out"=w26:errorcluster)  [unwired: 9 in]
      n186 = call "NI_USB6343_AO_Main_v2.vi"("error in (no error)"=w22, "VI Server Cluster"=w20) -> ("error out"=w23:errorcluster)  [unwired: 9 in]
      n187 = call "NI_USB6343_DAQmx_Counter_IN.vi"("error in (no error)"=w22, "VI Server Cluster"=w20) -> ("error out"=w25:errorcluster)  [unwired: 9 in]
      n188 = call "NI_USB6343_DAQmx_Counter_OUT.vi"("error in (no error)"=w22, "VI Server Cluster"=w20) -> ("error out"=w24:errorcluster)  [unwired: 9 in]
      n189 = call "NI_USB6343_Execute_Instructions_Processor.vi"("error in (no error)"=w22, "VI Server.RefsCluster"=w20) -> ("error out"=w21:errorcluster)  [unwired: 9 in]
      n190 = Build Array(w21, w24, w25, w23, w26, w30) -> (w27:errorcluster[])
      n191 = call "Merge Errors II.vi"("error array in"=w27, "error in 1 (no error)"=w29) -> ("error out.DUP"=w28:errorcluster)  [unwired: 4 in, 1 out]
    }
    frame Error {
    }
  }
  n192 = call-poly "VI Server_GetControl_Value_Ref.vi"("DataType"=tag "" ("DAQmx.Device"), "Control.Label"="DAQmx.Device", "error in"=w13, "SingleInstance"=TRUE, "VI Server.RefsCluster"=w11) -> ("error out"=w16:errorcluster, "Value"=w17:tag, "VI Server.RefsCluster.DUP"=w12:T2)  [unwired: 3 in, 1 out]
  n193 = call <vilib>:"DAQmx Reset Device.vi"("device in"=w17, "error in"=w16) -> ("error out"=w6:errorcluster)  [unwired: 13 in]
  n194 = call "Error _88709_DAQmx_Task Aborted or Device Not Present.vi"("Display Error Message"=FALSE, "error in"=w6) -> ("error out"=w5:errorcluster)  [unwired: 12 in, 1 out]
  n195 = call "VI Server_CloseRefs.vi"("error in"=w5, "VI Server.RefsCluster"=w12) -> ("error out"=w18:errorcluster)  [unwired: 9 in]
  n196 = call "NI_USB6343_Synch_CLOSE.vi"("error in"=w18) -> ("error out"=w9:errorcluster)  [unwired: 10 in]
  n197 = Current VI's Path() -> (path=w7:path)
  n198 = call "Close Window If in EXE mode.vi"("TopLevelVI Path"=w7, "error in"=w9) -> ("error out"=→"error out":errorcluster)  [unwired: 9 in]
